vi "Gamma Calcul.vi"(10 "Beta in":dbl format="%#_13g", 11 "Alpha in":dbl format="%#_13g") -> (2 "Gamma out":dbl)   [LabVIEW 2024, in "Game Board.lvclass"]
doc: "MIT Licence\nCopyright (c) 2024 David Grollier"
uses:
  Game Board.lvclass
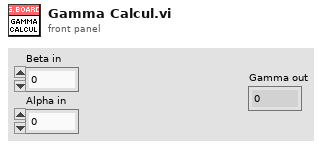
[diagram p1: front panel]
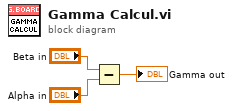
[diagram p0: block diagram]
diagram:
  n1 = Subtract(x="Beta in", y="Alpha in") -> (x-y=→"Gamma out":dbl)
